vi "07 - loading textures.vi"() -> ()   [LabVIEW 2015]
uses:
  Libraries/LibSDL2 Wrapper/Controls/Init Flags.ctl
  Libraries/LibSDL2 Wrapper/Controls/NULL.ctl
  Libraries/LibSDL2 Wrapper/LibSDL2.lvlib
  Libraries/LibSDL2_Image Wrapper/LibSDL2_Image.lvlib
  Libraries/SDL2 Utility/SDL2 Utility.lvlib
panel:
  out "Textures Per Second":dbl
  out "Error":string
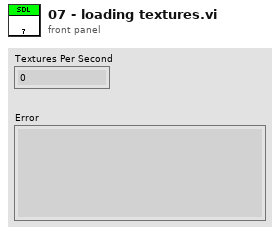
[diagram p1: front panel]
types:
  T1 = typedef "LibSDL2.lvlib/Init Flags.ctl" = u32
  T2 = typedef "LibSDL2.lvlib/NULL.ctl" = enum32{"NULL"}
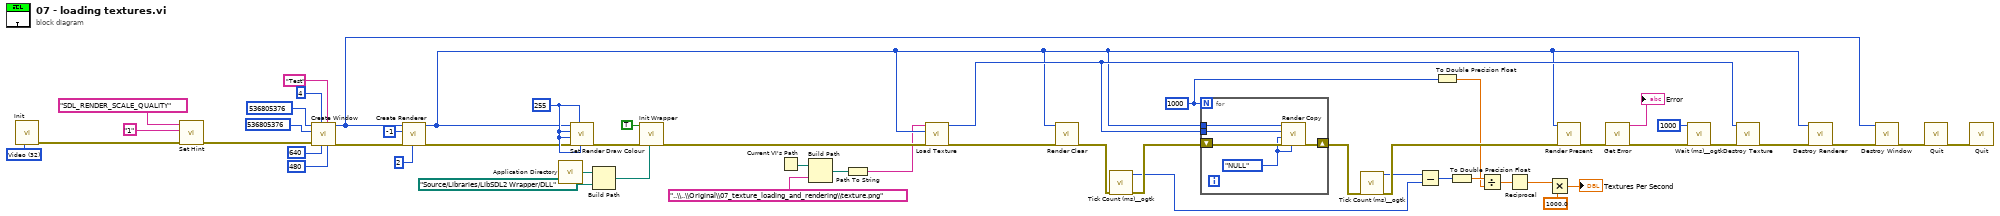
[diagram p0: block diagram]
diagram:
  w13 = 1000
  w33 = u8 255 ("R")
  w53 = T1 32 items=["Timer"=1, "Audio"=16, "Video"=32, "Joystick"=512, "Haptic"=4096, "Game Controller"=8192, "Events"=16384, "No Parachute"=1048576, "Everything"=17244689] ("Init Flags")
  n1 = call "Init.vi"("Flags"=w53) -> ("error out"=w41:errorcluster)  [unwired: 9 in, 1 out]
  n2 = call "Set Hint.vi"("error in"=w41, "Value"="1", "Name"="SDL_RENDER_SCALE_QUALITY") -> ("error out"=w40:errorcluster)  [unwired: 7 in, 1 out]
  n3 = call "Create Window.vi"("Height"=480, "Title"="Test", "Width"=640, "Flags"=u32 4, "error in"=w40, "Position y"=u32 536805376 ("Flags"), "Position x"=u32 536805376 ("Flags")) -> ("error out"=w37:errorcluster, "Window Pointer"=w36:u32)  [unwired: 3 in]
  n4 = call "Create Renderer.vi"("Flags"=u32 2, "error in"=w37, "Index"=-1, "Window Pointer"=w36) -> ("error out"=w26:errorcluster, "Renderer Pointer"=w27:u32)  [unwired: 6 in]
  n5 = call <vilib>:"Application Directory.vi"() -> ("Application Directory"=w6:path)
  n6 = call "Set Render Draw Colour.vi"("B"=w33, "A"=w33, "error in (no error)"=w26, "G"=w33, "R"=w33, "Renderer Pointer"=w27) -> ("error out"=w32:errorcluster)  [unwired: 4 in, 1 out]
  n7 = Build Path(base path=w6, name or relative path=path "Source/Libraries/LibSDL2 Wrapper/DLL" ("DLL Directory")) -> (appended path=w5:path)
  n8 = call "Init Wrapper.vi"("DLL Directory"=w5, "error in"=w32, "PNG (F)"=TRUE ("PNG")) -> ("error out"=w25:errorcluster)  [unwired: 7 in, 1 out]
  n9 = Current VI's Path() -> (path=w2:path)
  n10 = Build Path(base path=w2, name or relative path="..\\..\\Original\\07_texture_loading_and_rendering\\texture.png" ("File")) -> (appended path=w3:path)
  n11 = Path To String(path=w3) -> (string=w1:string)
  n12 = call "Load Texture.vi"("error in"=w25, "Renderer Pointer"=w27, "File"=w1) -> ("error out"=w24:errorcluster, "Optimised Texture Pointer"=w30:u32)  [unwired: 5 in, 2 out]
  n13 = call "Render Clear.vi"("error in"=w24, "Renderer Pointer"=w27) -> ("error out"=w21:errorcluster)  [unwired: 8 in, 1 out]
  n14 = call <userlib>:"Tick Count (ms)__ogtk.vi"("error in (no error)"=w21) -> ("error out"=w20:errorcluster, "millisecond timer value"=w16:u32)  [unwired: 9 in]
  n15 = for {
    N: w13 -> [_]
    tunnel: w30 -> [w58]
    tunnel: w27 -> [w57]
    shift-right: [w56] -> w19
    shift-left: w20 -> [w55]
    w54 = NULL."NULL" ("Null")
    n16 = call "Render Copy.vi"("Destination Rectangle Pointer"=w54, "error in"=w55, "Source Rectangle Pointer"=w54, "Texture Pointer"=w58, "Renderer Pointer"=w57) -> ("error out"=w56:errorcluster)  [unwired: 5 in, 1 out]
  }
  n17 = call <userlib>:"Tick Count (ms)__ogtk.vi"("error in (no error)"=w19) -> ("error out"=w18:errorcluster, "millisecond timer value"=w17:u32)  [unwired: 9 in]
  n18 = Subtract(x=w17, y=w16) -> (x-y=w15:u32)
  n19 = To Double Precision Float(number=w13) -> (double precision float=w12:dbl)
  n20 = To Double Precision Float(number=w15) -> (double precision float=w14:dbl)
  n21 = Divide(x=w14, y=w12) -> (x/y=w11:dbl)
  n22 = Reciprocal(x=w11) -> (1/x=w9:dbl)
  n23 = Multiply(x=w9, y=1000.0) -> (x*y=→"Textures Per Second":dbl)
  n24 = call "Render Present.vi"("error in"=w18, "Renderer Pointer"=w27) -> ("error out"=w23:errorcluster)  [unwired: 9 in]
  n25 = call "Get Error.vi"("error in"=w23) -> ("error out"=w22:errorcluster, "Error"=→"Error":string)  [unwired: 9 in]
  n26 = call <userlib>:"Wait (ms)__ogtk.vi"("error in (no error)"=w22, "milliseconds to wait"=u32 1000) -> ("error out"=w31:errorcluster)  [unwired: 8 in, 1 out]
  n27 = call "Destroy Texture.vi"("error in"=w31, "Texture Pointer"=w30) -> ("error out"=w29:errorcluster)  [unwired: 9 in]
  n28 = call "Destroy Renderer.vi"("error in"=w29, "Renderer Pointer"=w27) -> ("error out"=w28:errorcluster)  [unwired: 9 in]
  n29 = call "Destroy Window.vi"("error in"=w28, "Window Pointer"=w36) -> ("error out"=w44:errorcluster)  [unwired: 9 in]
  n30 = call "Quit.vi"("error in"=w44) -> ("error out"=w43:errorcluster)  [unwired: 10 in]
  n31 = call "Quit.vi"("error in"=w43) -> ()  [unwired: 10 in, 1 out]
